vi "Exercise1.25-QueneTest.vi"() -> ()   [LabVIEW 2013]
panel:
  out "RandOut":dbl(graph)
  out "RandIn":dbl(graph)
  out "Numeric":i32
  out "elements in queue":i32
  in  "stop":bool
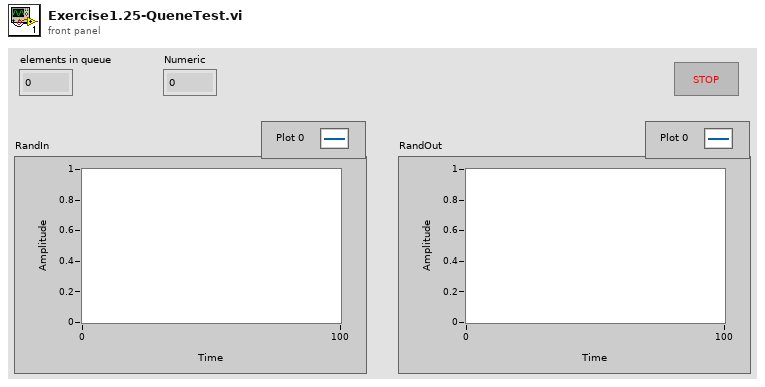
[diagram p1: front panel]
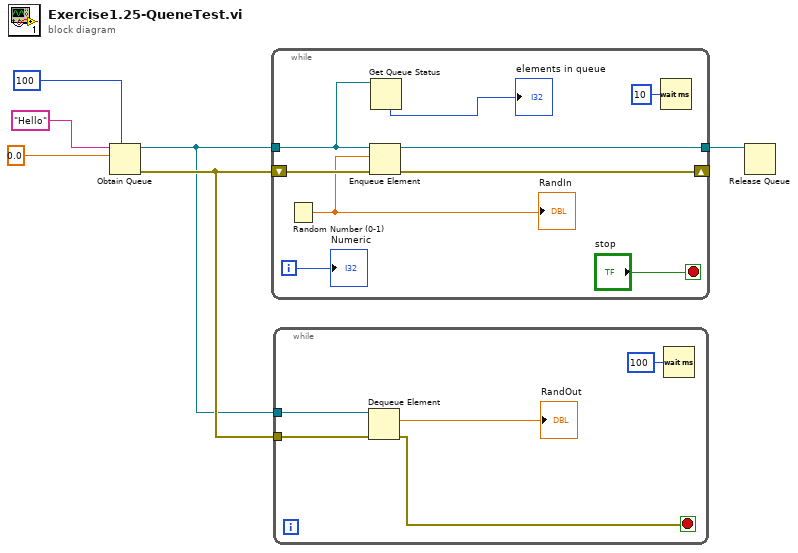
[diagram p0: block diagram]
diagram:
  n1 = Obtain Queue(max queue size (-1, unlimited)=100, name (unnamed)="Hello", element data type=0.0) -> (queue out=w1:refnum<queue>, error out=w2:errorcluster)  [unwired: 2 in, 1 out]
  n2 = while {
    tunnel: w1 -> [w13]
    tunnel: [w15] -> w3
    shift-right: [w9] -> _
    shift-left: w2 -> [w10]
    i -> [w12]
    stop <- "stop" stop-if-true
    n3 = Random Number (0-1)() -> (number: 0 to 1=w7:dbl)
    "RandIn" <- w7
    n4 = Enqueue Element(queue=w13, element=w7, error in (no error)=w10) -> (queue out=w15:refnum<queue>, error out=w9:errorcluster)  [unwired: 1 in, 1 out]
    n5 = Get Queue Status(queue=w13) -> (# elements in queue=→"elements in queue":i32)  [unwired: 2 in, 7 out]
    n6 = Wait (ms)(milliseconds to wait=u32 10) -> ()  [unwired: 1 out]
    "Numeric" <- w12
  }
  n7 = while {
    tunnel: w1 -> [w20]
    tunnel: w2 -> [w18]
    stop <- w17 stop-if-true
    n8 = Dequeue Element(queue=w20, error in (no error)=w18) -> (element=→"RandOut":dbl, error out=w17:errorcluster)  [unwired: 1 in, 2 out]
    n9 = Wait (ms)(milliseconds to wait=u32 100) -> ()  [unwired: 1 out]
  }
  n10 = Release Queue(queue=w3) -> ()  [unwired: 2 in, 3 out]
